vi "Image.vi"(2 "XRef":refnum<vi>, 3 "State In":T1) -> (0 "Image":picture)   [LabVIEW 2015, in "Async-And-Forget.xnode"]
doc: "This ability VI is used to describe your XNode's appearance. The origin of Image corresponds to the top-left corner of your XNode. The bounds of your XNode are used to crop this image. If you want LabVIEW to update your image, you need to inform it through the UpdateImage or UpdateImageAndBounds replies. Any areas where you do not draw are transparent, so regions intended to appear white should be explicitly drawn.\n \n Remember to localize any strings that are part of your image.\n\nDefault behavior: None.\n\nThis ability does not provide UI and OS messages are not handled."
uses:
  Async-And-Forget.xnode
  State.ctl
  <vilib>/Utility/miscctls.llb/LVRectTypeDef.ctl
  <vilib>/picture/picture.llb/imagedata.ctl
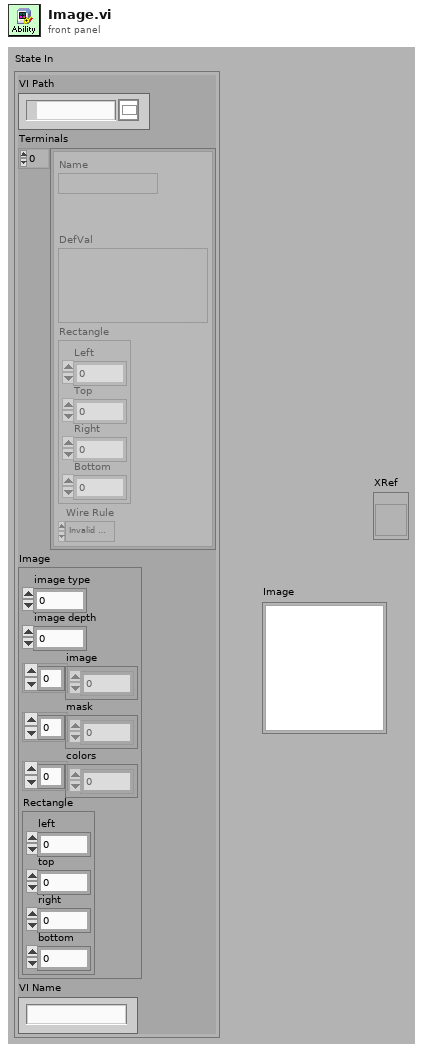
[diagram p1: front panel]
types:
  T1 = typedef "Async-And-Forget.xnode/State.ctl" = cluster{"VI Path":path, "Terminals":cluster{"Name":string, "DefVal":variant, "Rectangle":T2, "Wire Rule":enum16{"Invalid Wire Rule", "Required", "Recommended", "Optional", "Dynamic Dispatch"}}[], "Image":T3, "VI Name":string}
  T2 = typedef "LVRectTypeDef.ctl" = cluster{"Left":i16, "Top":i16, "Right":i16, "Bottom":i16}
  T3 = typedef "imagedata.ctl" = cluster{"image type":i32, "image depth":i32, "image":u8[], "mask":u8[], "colors":u32[], "Rectangle":cluster{"left":i16, "top":i16, "right":i16, "bottom":i16}}
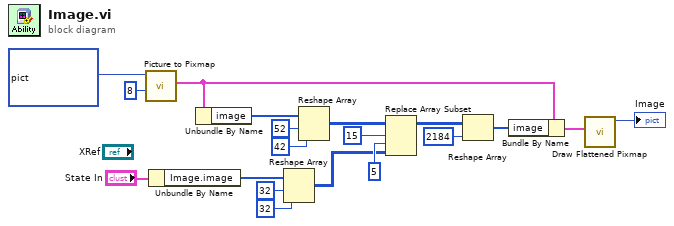
[diagram p0: block diagram]
diagram:
  n1 = call <vilib>:"Picture to Pixmap.vi"("depth"=8, "picture"=picture bytes[6894] ("Image")) -> ("image data"=w10:T3)  [unwired: 8 in, 1 out]
  n2 = Unbundle By Name("State In") -> ("Image.image"=w6:u8[])
  n3 = Unbundle By Name(w10) -> ("image"=w7:u8[])
  n4 = Reshape Array(w6, 32 ("dimension size"), 32 ("dimension size")) -> (w11:u8[][])
  n5 = Reshape Array(w7, 52 ("dimension size"), 42 ("dimension size")) -> (w14:u8[][])
  n6 = Replace Array Subset(array=w14, new element=w11, index (row)=15 ("disabled index (row)"), index (col)=5 ("index (row)")) -> (w5:u8[][])
  n7 = Reshape Array(w5, 2184 ("dimension size")) -> (w4:u8[])
  n8 = Bundle By Name(cluster=w10, "image"=w4) -> (w2:T3)
  n9 = call <vilib>:"Draw Flattened Pixmap.vi"("image data"=w2) -> ("new picture"=→"Image":picture)  [unwired: 8 in]
